vi "Read Value.vi"(8 "error in (no error)":errorcluster, 11 "1D wfm (DBL) Result in":refnum<class "1D wfm (DBL) Result.lvclass">) -> (0 "error out":errorcluster, 2 "Value":dbl, 3 "1D wfm (DBL) Result out":refnum<class "1D wfm (DBL) Result.lvclass">)   [LabVIEW 2015, in "1D wfm (DBL) Result.lvclass"]
uses:
  1D wfm (DBL) Result.lvclass
  1D wfm (DBL) Result.lvclass/1D wfm (DBL) Result.ctl
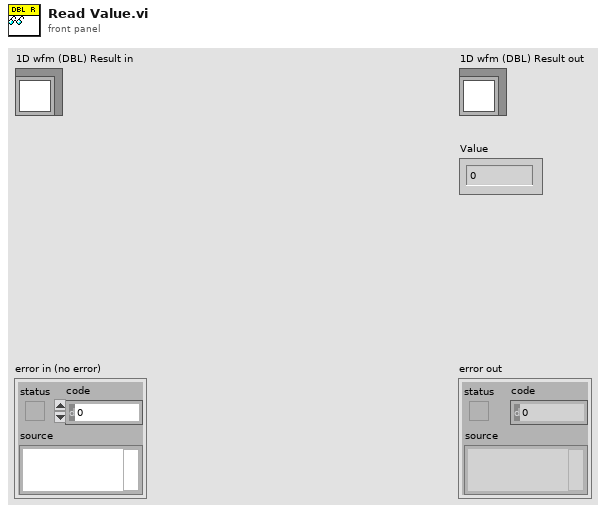
[diagram p1: front panel]
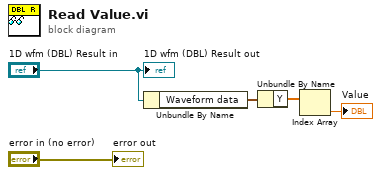
[diagram p0: block diagram]
diagram:
  n1 = Unbundle By Name("1D wfm (DBL) Result in") -> ("Waveform data"=w4:waveform(dbl))
  n2 = Unbundle By Name(w4) -> ("Y"=w3:dbl[])
  n3 = Index Array(array=w3) -> (element=→"Value":dbl)  [unwired: 1 in]
  "error out" <- "error in (no error)"
  "1D wfm (DBL) Result out" <- "1D wfm (DBL) Result in"
